vi "Timer_Test.vi"(8 "error in (no error)":errorcluster) -> (0 "error out":errorcluster)   [LabVIEW 2019, in "Data_Logger.lvlib"]
uses:
  Data_Logger.lvlib
panel:
  out "concatenated string":string
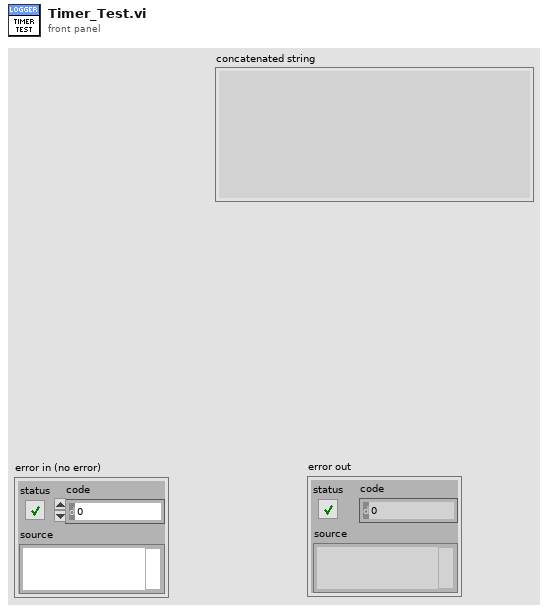
[diagram p1: front panel]
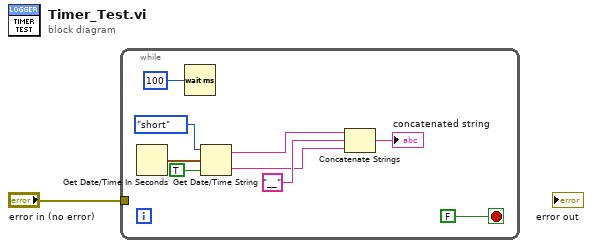
[diagram p0: block diagram]
diagram:
  n1 = while {
    tunnel: "error in (no error)" -> [_]
    stop <- FALSE stop-if-true
    n2 = Get Date/Time In Seconds() -> (seconds since 1Jan1904=w9:timestamp)
    n3 = Wait (ms)(milliseconds to wait=u32 100) -> ()  [unwired: 1 out]
    n4 = Get Date/Time String(date format (0)=enum16{"short", "long", "abbreviated"}."short", seconds (now)=w9, want seconds? (F)=TRUE) -> (date string=w5:string, time string=w4:string)
    n5 = Concatenate Strings(w5, "__", w4) -> (→"concatenated string":string)
  }
